vi "KE2260B Configure Output Mode.vi"(8 "error in (no error)":errorcluster, 10 "Output Mode ( 0 : CVHS )":enum16{"CVHS", "CCHS", "CVLS", "CCLS"}(ring) caption="Output Mode", 11 "VISA resource name":refnum<visa-resource-name>) -> (0 "error out":errorcluster, 3 "VISA resource name out":refnum<visa-resource-name>)   [LabVIEW 2021, in "Keithley 2260B.lvlib"]
doc: "Configures High Speed Priority, or Slew Rate Priority CV or CC mode."
uses:
  Keithley 2260B.lvlib
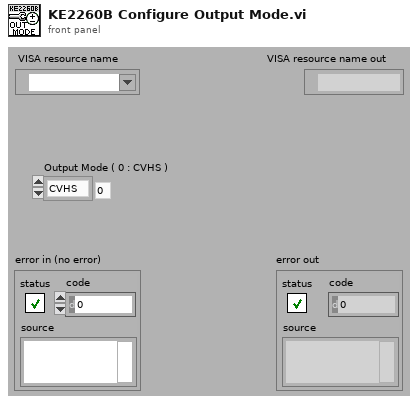
[diagram p1: front panel]
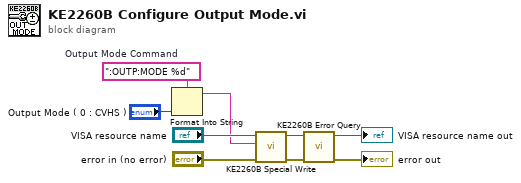
[diagram p0: block diagram]
diagram:
  w7 = ":OUTP:MODE %d"  # Output Mode Command
  n1 = Format Into String(format string=w7, "Output Mode ( 0 : CVHS )") -> (resulting string=w2:string)  [unwired: 2 in, 1 out]
  n2 = call "KE2260B Special Write.vi"("error in (no error)"="error in (no error)", "Write Buffer (\"\")"=w2, "VISA session"="VISA resource name") -> ("error out"=w6:errorcluster, "dup VISA session"=w5:refnum<visa-resource-name>)  [unwired: 6 in, 1 out]
  n3 = call "KE2260B Error Query.vi"("error in (no error)"=w6, "VISA resource name"=w5) -> ("error out"=→"error out":errorcluster, "VISA resource name out"=→"VISA resource name out":refnum<visa-resource-name>)  [unwired: 6 in, 2 out]
